vi "Scale wForms for wave file.vi"(0 "Signal IN":waveform(dbl)[](array[waveform]), 7 "Desired Level (EU)":dbl=1.0) -> (13 "Ref Label":string, 14 "Signal OUT":waveform(dbl)[](array[waveform]))   [LabVIEW 2020, in "WaveFile.lvclass"]
uses:
  WaveFile.lvclass
  API/GSwFormDSP_class/GSwFormDSP.lvclass
panel:
  # "0dB will force maximum scale!"
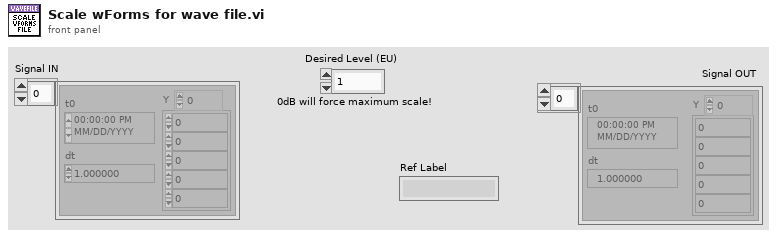
[diagram p1: front panel]
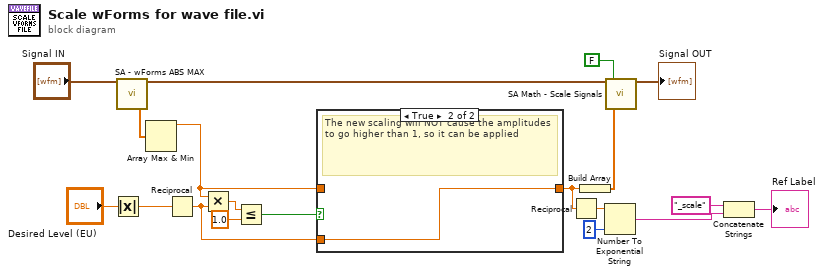
[diagram p0: block diagram]
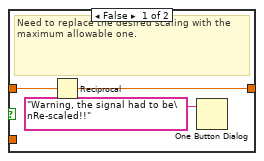
[diagram p2: hidden frame]
diagram:
  n1 = Absolute Value(x="Desired Level (EU)") -> (abs(x)=w8:dbl)
  n2 = call "SA - wForms ABS MAX.vi"("wForms IN"="Signal IN") -> ("ABS MAX's"=w2:dbl[], "wForms OUT"=w3:waveform(dbl)[])  [unwired: 17 in]
  n3 = Array Max & Min(array=w2) -> (max value=w1:dbl)  [unwired: 3 out]
  n4 = Reciprocal(x=w8) -> (1/x=w14:dbl)
  n5 = Multiply(x=w1, y=w14) -> (x*y=w15:dbl)
  n6 = Less Or Equal?(x=w15, y=1.0) -> (x <= y?=w17:bool)
  n7 = case shown="True" w17 {
    tunnel: w14 -> [_ w23]
    tunnel: [w21 w23] -> w11
    tunnel: w1 -> [w22 _]
    frame False {
      # "Need to replace the desired scaling with the maximum allowable one."
      n8 = Reciprocal(x=w22) -> (1/x=w21:dbl)
      n9 = One Button Dialog(message="Warning, the signal had to be\nRe-scaled!!") -> ()  [unwired: 1 in, 1 out]
    }
    frame True {
      # "The new scaling will NOT cause the amplitudes to go higher than 1, so it can be applied"
    }
  }
  n10 = Reciprocal(x=w11) -> (1/x=w5:dbl)
  n11 = Build Array(w11) -> (w12:dbl[])
  n12 = Number To Exponential String(number=w5, precision (6)=i16 2) -> (E-format string=w6:string)  [unwired: 2 in]
  n13 = call "SA Math - Scale Signals.vi"("Signal IN"=w3, "Anotate Signal Name"=FALSE, "Scaling Factors"=w12) -> ("Signal OUT"=→"Signal OUT":waveform(dbl)[])  [unwired: 15 in, 1 out]
  n14 = Concatenate Strings("_scale", w6) -> (→"Ref Label":string)
